vi "Add Output.vi"(0 "PainOutputTerminal in":refnum<class "SystemLinkOutputTerminal.lvclass">, 5 "Comiplation message":T1[](array[typedef]), 11 "error in (no error)":errorcluster) -> (4 "PainOutputTerminal out":refnum<class "SystemLinkOutputTerminal.lvclass">, 15 "error out":errorcluster)   [LabVIEW 2016, in "SystemLinkOutputTerminal.lvclass"]
uses:
  SystemLinkOutputTerminal.lvclass
  common/function utils/Validate_message.ctl
  common/function utils/Validate_MessageStatus.ctl
  Plain OT/PainOutputTerminal.lvclass
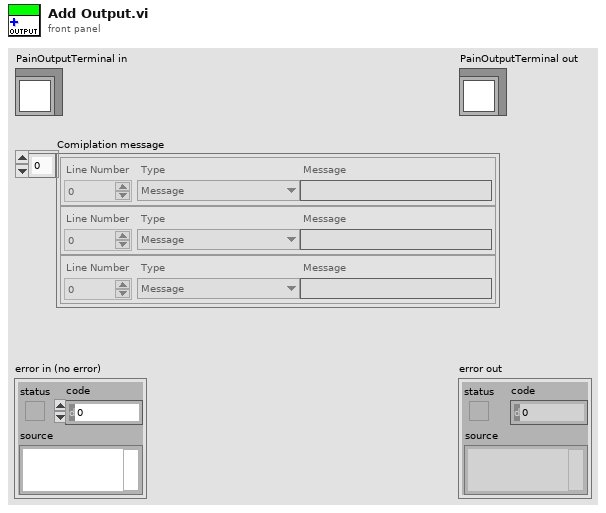
[diagram p1: front panel]
types:
  T1 = typedef "Validate_message.ctl" = cluster{"Line Number":i64, "Type":T2, "Message":string}
  T2 = typedef "Validate_MessageStatus.ctl" = enum16{"Message", "Warning", "Error"}
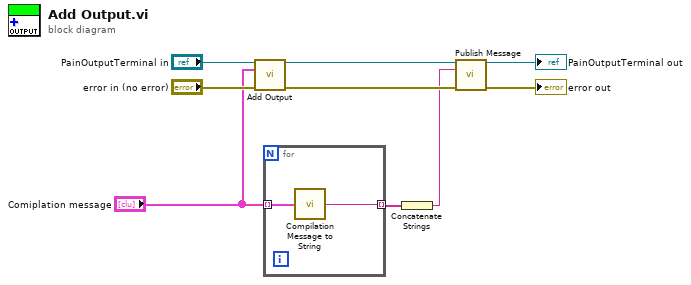
[diagram p0: block diagram]
diagram:
  n1 = call-parent "Add Output.vi"("PainOutputTerminal in"="PainOutputTerminal in", "Comiplation message"="Comiplation message", "error in (no error)"="error in (no error)") -> ("PainOutputTerminal out"=w8:refnum<class "SystemLinkOutputTerminal.lvclass">, "error out"=w9:errorcluster)  [unwired: 11 in]
  n2 = for {
    tunnel: "Comiplation message" -> [w11] mode=indexing
    tunnel: [w10] -> w2 mode=indexing
    n3 = call "Compilation Message to String.vi"("Message"=w11) -> ("Messgae"=w10:string)  [unwired: 4 in]
  }
  n4 = Concatenate Strings(w2) -> (w1:string)
  n5 = call "Publish Message.vi"("SystemLinkOutputTerminal in"=w8, "Publish Message"=w1, "error in (no error)"=w9) -> ("SystemLinkOutputTerminal out"=→"PainOutputTerminal out":refnum<class "SystemLinkOutputTerminal.lvclass">, "error out"=→"error out":errorcluster)  [unwired: 11 in]
